vi "FTW-Logger-SerializeEvent.vi"(0 "Event Type":string, 5 "Event Data":string, 7 "Source (unwired for call chain, Empty to omit)":string="CallChain", 11 "Error to Log":errorcluster) -> (4 "Serialized Event":string)   [LabVIEW 2013, in "FTW-Logger.lvclass"]
uses:
  FTW-Logger.lvclass
panel:
  # "Inputs"
  # "Outputs"
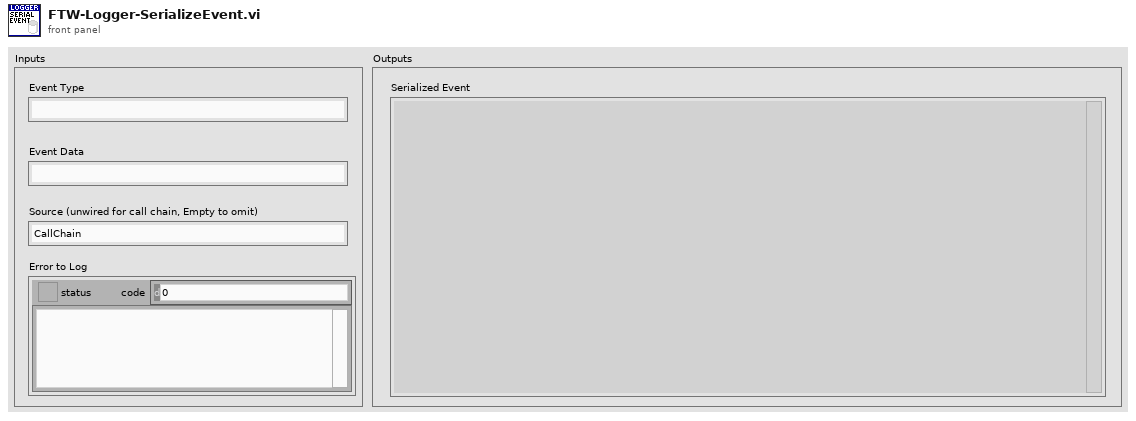
[diagram p1: front panel]
types:
  T1 = typedef "FTW-Event.ctl" = cluster{"Count":i32, "Uptime":dbl, "Timestamp":string, "Source":string, "Type":string, "Data":string, "Error":errorcluster}
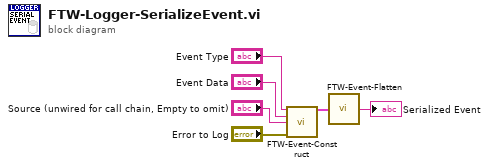
[diagram p0: block diagram]
diagram:
  n1 = call "FTW-Event-Construct.vi"("Event Type"="Event Type", "Event Data"="Event Data", "Source"="Source (unwired for call chain, Empty to omit)", "Error to Log"="Error to Log") -> ("Event"=w2:T1)  [unwired: 11 in]
  n2 = call "FTW-Event-Flatten.vi"("Event"=w2) -> ("Flattened Event"=→"Serialized Event":string)  [unwired: 14 in]
